vi "Bundle control and indicator references.vi"(8 "error in":errorcluster, 11 "UI elements cluster":T1) -> (0 "error out":errorcluster, 3 "UI elements cluster":T1)   [LabVIEW 2013]
uses:
  Typedefs/UI ctrl refs cluster.ctl
  Typedefs/Laser control knob.ctl
  Typedefs/Frame Size.ctl
  Typedefs/Plane Mode.ctl
  Typedefs/PMT control knob.ctl
  Global Variables/gl_UI Ctrl Refs.vi
panel:
  out "Ctrl ref names in typedef cluster":string[](array[string])
  out "Dynamically acquired UI element names":string[](array[string])
  out "IP same as OP?":T2
  out "Errors":errorcluster[](array[cluster])
  out "UI element names and status":cluster{"Label.Text":string, "Found":bool}[](array[cluster])
  # "<----- If the LED is off for a UI element it means that that this VI fails to acquire its reference correctly. In that case upgrade this VI to handle that element."
  # "The top 5 should be the same.\nThe rest should be updated so not the same."
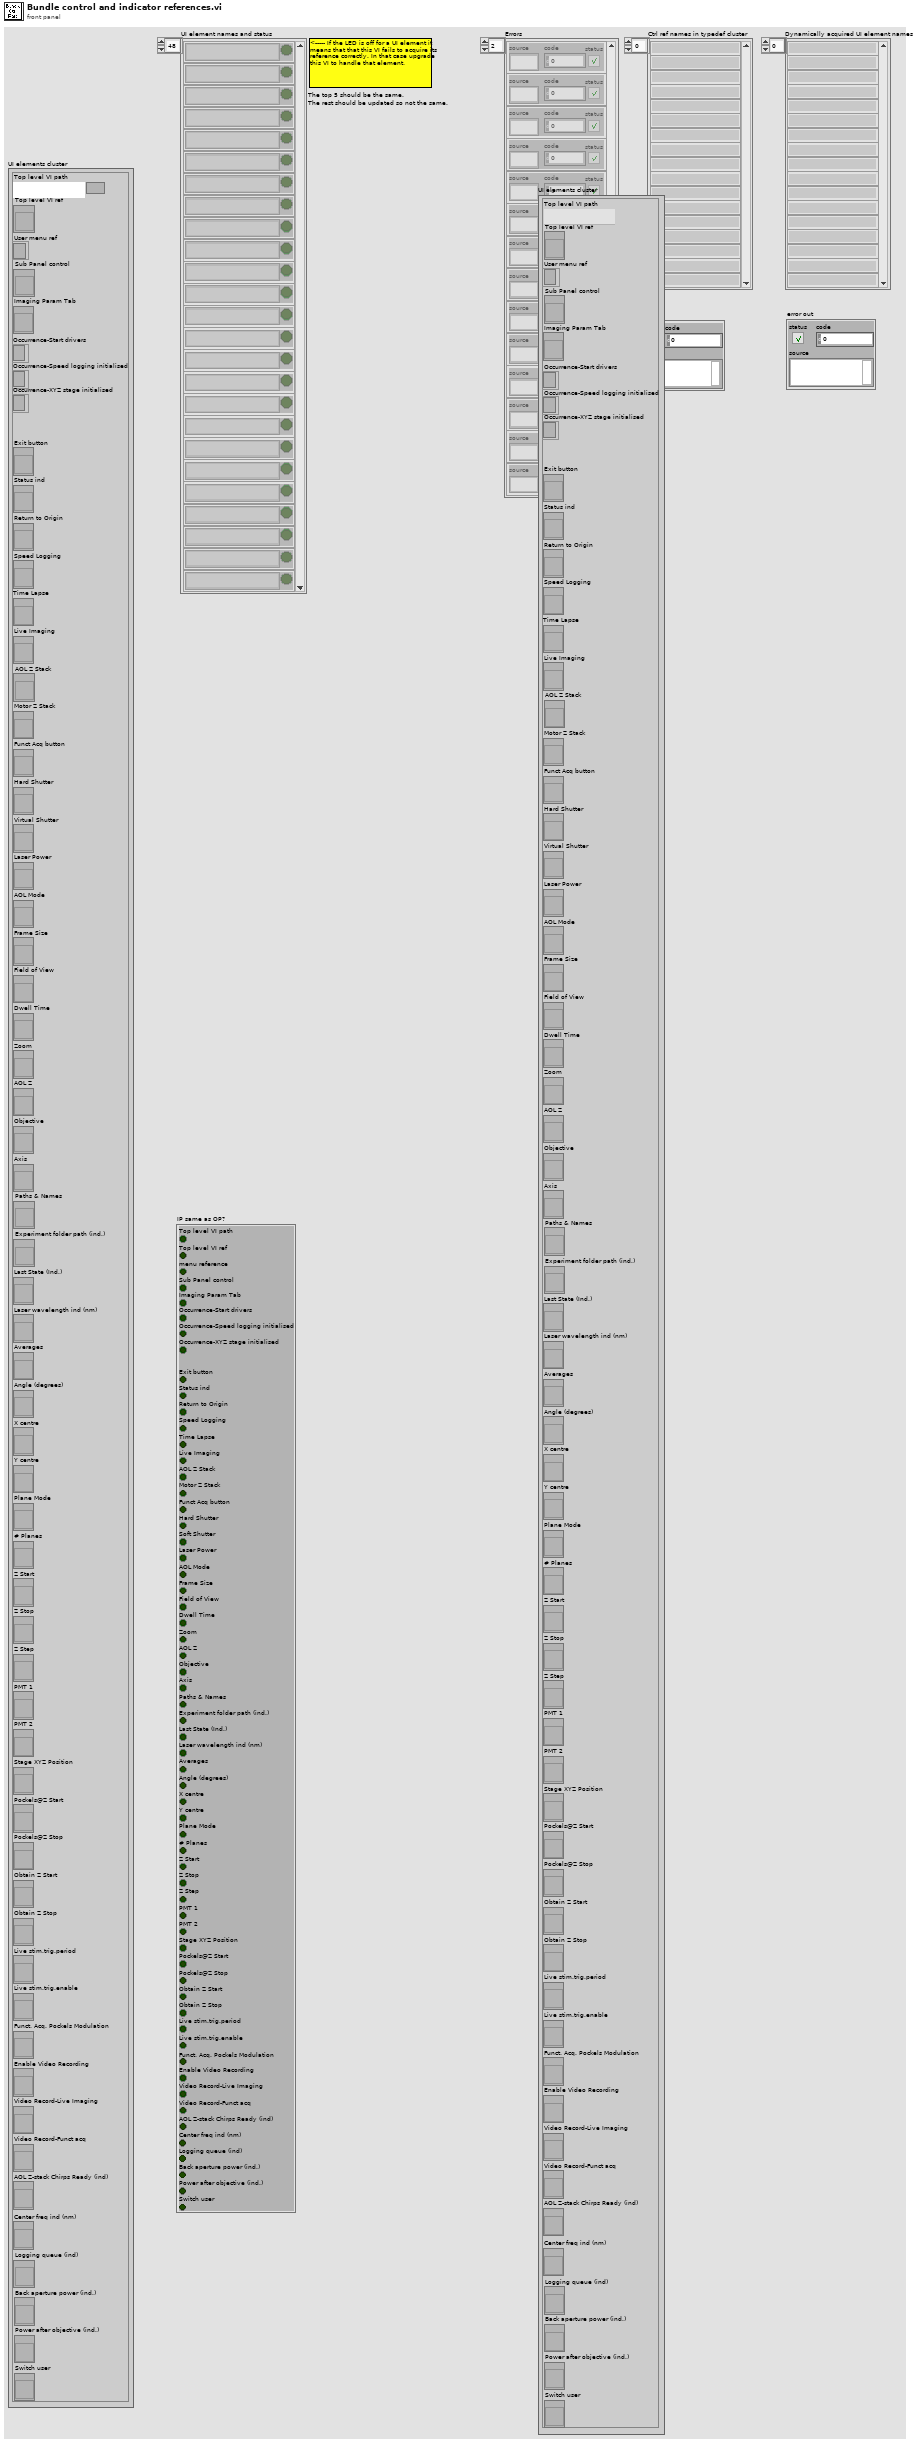
[diagram p1: front panel]
types:
  T1 = typedef "UI ctrl refs cluster.ctl" = cluster{"Top level VI path":path, "Top level VI ref":refnum<vi>, "User menu ref":refnum<k9>, "Sub Panel control":refnum<vi>, "Imaging Param Tab":refnum<vi>, "Occurrence-Start drivers":refnum<k4>, "Occurrence-Speed logging initialised":refnum<k4>, "Occurrence-XYZ stage initialised":refnum<k4>, "Exit button":refnum<vi>, "Status ind":refnum<vi>, "Return to Origin":refnum<vi>, "Speed Logging":refnum<vi>, "Time Lapse":refnum<vi>, "Live Imaging":refnum<vi>, "AOL Z Stack":refnum<vi>, "Motor Z Stack":refnum<vi>, "Funct Acq button":refnum<vi>, "Hard Shutter":refnum<vi>, "Virtual Shutter":refnum<vi>, "Laser Power":refnum<vi>, "AOL Mode":refnum<vi>, "Frame Size":refnum<vi>, "Field of View":refnum<vi>, "Dwell Time":refnum<vi>, "Zoom":refnum<vi>, "AOL Z":refnum<vi>, "Objective":refnum<vi>, "Axis":refnum<vi>, "Paths & Names":refnum<vi>, "Experiment folder path (ind.)":refnum<vi>, "Last State (Ind.)":refnum<vi>, "Laser wavelength ind (nm)":refnum<vi>, "Averages":refnum<vi>, "Angle (degrees)":refnum<vi>, "X centre":refnum<vi>, "Y centre":refnum<vi>, "Plane Mode":refnum<vi>, "# Planes":refnum<vi>, "Z Start":refnum<vi>, "Z Stop":refnum<vi>, "Z Step":refnum<vi>, "PMT 1":refnum<vi>, "PMT 2":refnum<vi>, "Stage XYZ Position":refnum<vi>, "Pockels@Z Start":refnum<vi>, "Pockels@Z Stop":refnum<vi>, "Obtain Z Start":refnum<vi>, "Obtain Z Stop":refnum<vi>, "Live stim.trig.period":refnum<vi>, "Live stim.trig.enable":refnum<vi>, "Funct. Acq. Pockels Modulation":refnum<vi>, "Enable Video Recording":refnum<vi>, "Video Record-Live Imaging":refnum<vi>, "Video Record-Funct acq":refnum<vi>, "AOL Z-stack Chirps Ready (ind)":refnum<vi>, "Center freq ind (nm)":refnum<vi>, "Logging queue (ind)":refnum<vi>, "Back aperture power (ind.)":refnum<vi>, "Power after objective (ind.)":refnum<vi>, "Switch user":refnum<vi>}
  T2 = cluster{"Top level VI path":bool, "Top level VI ref":bool, "menu reference":bool, "Sub Panel control":bool, "Imaging Param Tab":bool, "Occurrence-Start drivers":bool, "Occurrence-Speed logging initialised":bool, "Occurrence-XYZ stage initialised":bool, "Exit button":bool, "Status ind":bool, "Return to Origin":bool, "Speed Logging":bool, "Time Lapse":bool, "Live Imaging":bool, "AOL Z Stack":bool, "Motor Z Stack":bool, "Funct Acq button":bool, "Hard Shutter":bool, "Soft Shutter":bool, "Laser Power":bool, "AOL Mode":bool, "Frame Size":bool, "Field of View":bool, "Dwell Time":bool, "Zoom":bool, "AOL Z":bool, "Objective":bool, "Axis":bool, "Paths & Names":bool, "Experiment folder path (ind.)":bool, "Last State (Ind.)":bool, "Laser wavelength ind (nm)":bool, "Averages":bool, "Angle (degrees)":bool, "X centre":bool, "Y centre":bool, "Plane Mode":bool, "# Planes":bool, "Z Start":bool, "Z Stop":bool, "Z Step":bool, "PMT 1":bool, "PMT 2":bool, "Stage XYZ Position":bool, "Pockels@Z Start":bool, "Pockels@Z Stop":bool, "Obtain Z Stop":bool, "Obtain Z Start":bool, "Live stim.trig.period":bool, "Live stim.trig.enable":bool, "Funct. Acq. Pockels Modulation":bool, "Enable Video Recording":bool, "Video Record-Live Imaging":bool, "Video Record-Funct acq":bool, "AOL Z-stack Chirps Ready (ind)":bool, "Center freq ind (nm)":bool, "Logging queue (ind)":bool, "Back aperture power (ind.)":bool, "Power after objective (ind.)":bool, "Switch user":bool}
  T3 = cluster{"Top level VI path":bool, "Top level VI ref":bool, "User menu ref":bool, "Sub Panel control":bool, "Imaging Param Tab":bool, "Occurrence-Start drivers":bool, "Occurrence-Speed logging initialised":bool, "Occurrence-XYZ stage initialised":bool, "Exit button":bool, "Status ind":bool, "Return to Origin":bool, "Speed Logging":bool, "Time Lapse":bool, "Live Imaging":bool, "AOL Z Stack":bool, "Motor Z Stack":bool, "Funct Acq button":bool, "Hard Shutter":bool, "Virtual Shutter":bool, "Laser Power":bool, "AOL Mode":bool, "Frame Size":bool, "Field of View":bool, "Dwell Time":bool, "Zoom":bool, "AOL Z":bool, "Objective":bool, "Axis":bool, "Paths & Names":bool, "Experiment folder path (ind.)":bool, "Last State (Ind.)":bool, "Laser wavelength ind (nm)":bool, "Averages":bool, "Angle (degrees)":bool, "X centre":bool, "Y centre":bool, "Plane Mode":bool, "# Planes":bool, "Z Start":bool, "Z Stop":bool, "Z Step":bool, "PMT 1":bool, "PMT 2":bool, "Stage XYZ Position":bool, "Pockels@Z Start":bool, "Pockels@Z Stop":bool, "Obtain Z Start":bool, "Obtain Z Stop":bool, "Live stim.trig.period":bool, "Live stim.trig.enable":bool, "Funct. Acq. Pockels Modulation":bool, "Enable Video Recording":bool, "Video Record-Live Imaging":bool, "Video Record-Funct acq":bool, "AOL Z-stack Chirps Ready (ind)":bool, "Center freq ind (nm)":bool, "Logging queue (ind)":bool, "Back aperture power (ind.)":bool, "Power after objective (ind.)":bool, "Switch user":bool}
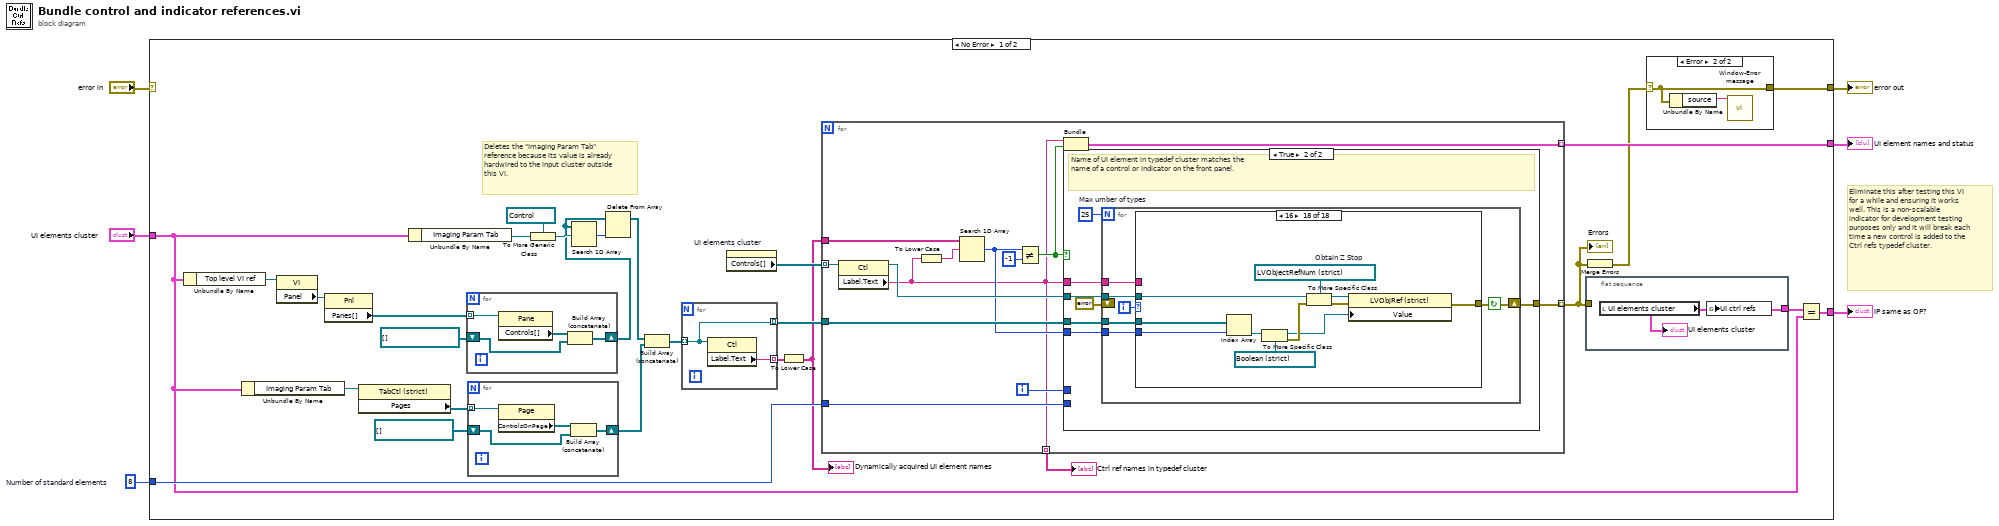
[diagram p0: block diagram]
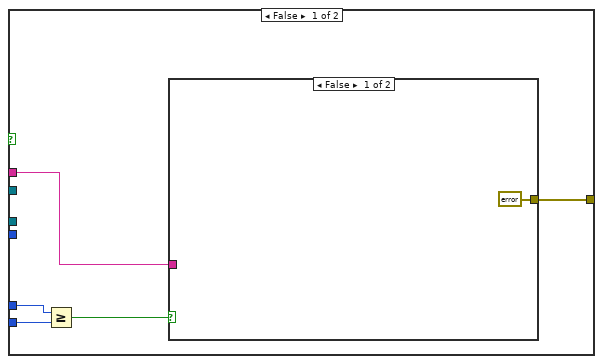
[diagram p3: hidden frame]
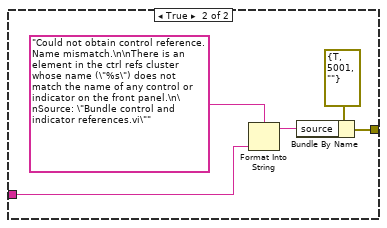
[diagram p4: hidden frame]
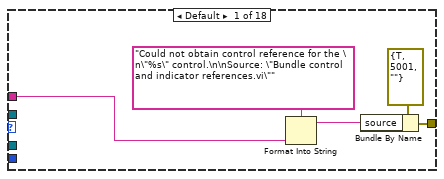
[diagram p5: hidden frame]
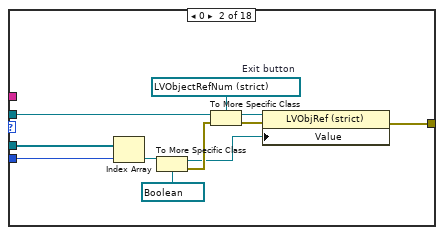
[diagram p6: hidden frame]
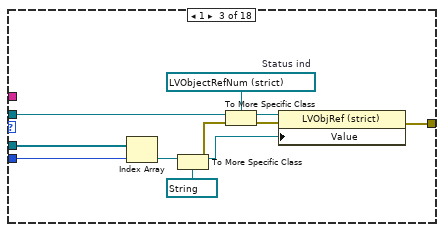
[diagram p7: hidden frame]
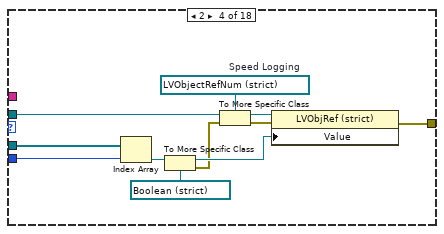
[diagram p8: hidden frame]
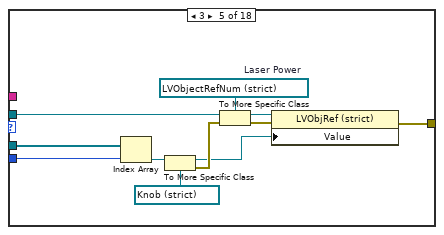
[diagram p9: hidden frame]
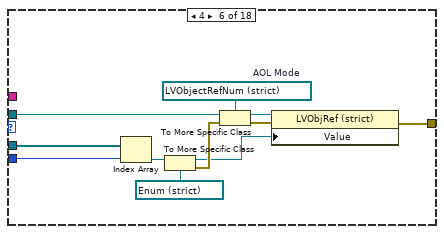
[diagram p10: hidden frame]
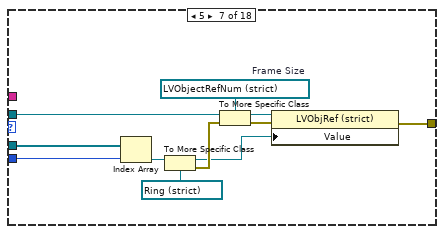
[diagram p11: hidden frame]
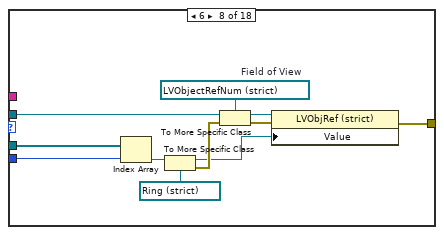
[diagram p12: hidden frame]
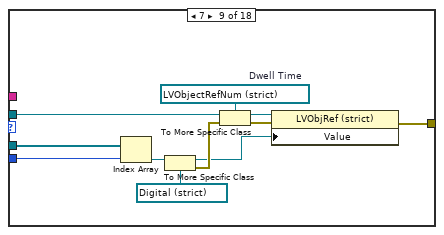
[diagram p13: hidden frame]
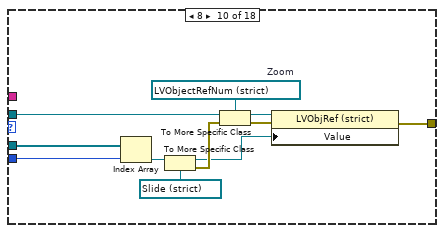
[diagram p14: hidden frame]
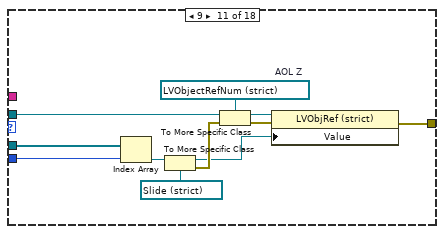
[diagram p15: hidden frame]
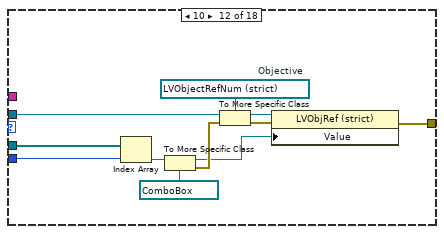
[diagram p16: hidden frame]
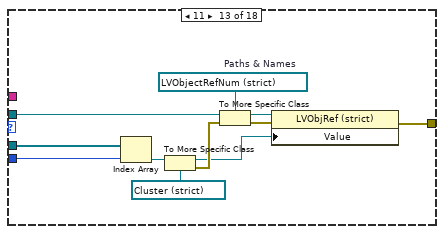
[diagram p17: hidden frame]
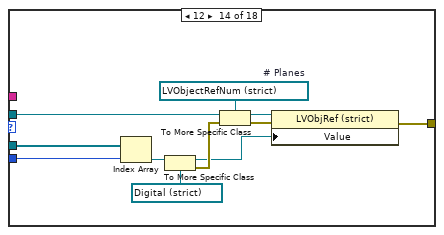
[diagram p18: hidden frame]
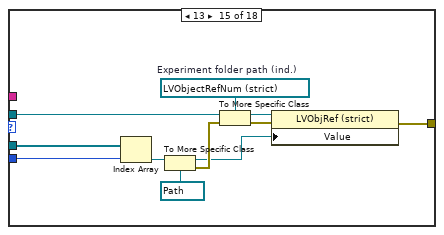
[diagram p19: hidden frame]
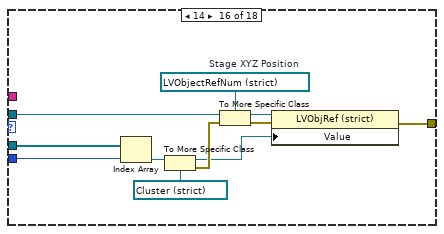
[diagram p20: hidden frame]
diagram:
  w2 = 8  # Number of standard elements
  # "Eliminate this after testing this VI for a while and ensuring it works well. This is a non-scalable indicator for development testing purposes only and it will break each time a new control is added to the Ctrl refs typedef cluster."
  n1 = case shown="No Error" "error in" {
    selector: "error in" -> [_ w277]
    tunnel: [w24 _] -> w6
    tunnel: "UI elements cluster" -> [w10 _]
    tunnel: [w22 _] -> w1
    tunnel: [w13 w277] -> w3
    tunnel: w2 -> [w12 _]
    frame No Error {
      # "Deletes the \"Imaging Param Tab\" reference because its value is already hardwired to the input cluster outside this VI."
      n2 = Unbundle By Name(w10) -> ("Top level VI ref"=w33:refnum<vi>)
      n3 = Unbundle By Name(w10) -> ("Imaging Param Tab"=w19:refnum<vi>)
      n4 = property on="Property Node" class="VI"(reference=w33) -> ("Panel"=w34:refnum<vi>)  [unwired: 1 in, 2 out]
      n5 = property on="Property Node" class="Pnl"(reference=w34) -> ("Panes[]"=w31:refnum<vi>[])  [unwired: 1 in, 2 out]
      n6 = property on="Property Node" class="TabCtl (strict)"(reference=w19) -> ("Pages"=w30:refnum<vi>[])  [unwired: 1 in, 2 out]
      n7 = Unbundle By Name(w10) -> ("Imaging Param Tab"=w11:refnum<vi>)
      n8 = for {
        shift-right: [w275] -> w9
        shift-left: refnum<vi>[] [] -> [w274]
        tunnel: w31 -> [w273] mode=indexing
        n9 = property class="Pane"(reference=w273) -> ("Controls[]"=w276:refnum<vi>[])  [unwired: 1 in, 2 out]
        n10 = Build Array (concatenate)(w276, w274) -> (w275:refnum<vi>[])
      }
      n11 = for {
        shift-right: [w269] -> w28
        shift-left: refnum<vi>[] [] -> [w268]
        tunnel: w30 -> [w267] mode=indexing
        n12 = property class="Page"(reference=w267) -> ("ControlsOnPage"=w270:refnum<vi>[])  [unwired: 1 in, 2 out]
        n13 = Build Array (concatenate)(w270, w268) -> (w269:refnum<vi>[])
      }
      n14 = To More Generic Class(target class=refnum<vi> refnum ("element"), reference=w11) -> (generic class reference=w18:refnum<vi>)
      n15 = Search 1D Array(1D array=w9, element=w18) -> (index of element=w16:i32)  [unwired: 1 in]
      n16 = Delete From Array(array=w9, index=w16) -> (array with subset deleted=w15:refnum<vi>[])  [unwired: 1 in, 1 out]
      n17 = Build Array (concatenate)(w15, w28) -> (w27:refnum<vi>[])
      n18 = for {
        tunnel: w27 -> [w271] mode=indexing
        tunnel: [w272] -> w25 mode=indexing
        tunnel: [w271] -> w23 mode=indexing
        n19 = property on="Property Node" class="Ctl"(reference=w271) -> ("Label.Text"=w272:string)  [unwired: 1 in, 2 out]
      }
      n20 = property on="UI elements cluster" class="Clust (strict)"() -> ("Controls[]"=w26:refnum<vi>[])  [unwired: 2 in, 2 out]
      n21 = To Lower Case(string=w25) -> (all lower case string=w8:string[])
      "Dynamically acquired UI element names" <- w8
      n22 = for {
        tunnel: w26 -> [w50] mode=indexing
        tunnel: w8 -> [w49]
        tunnel: [w47] -> w24 mode=indexing
        tunnel: [w45] -> w21 mode=indexing
        tunnel: w23 -> [w43]
        tunnel: w12 -> [w40]
        tunnel: [w38] -> w7 mode=indexing
        i -> [w41]
        n23 = property on="Property Node" class="Ctl"(reference=w50) -> (reference out=w46:refnum<vi>, "Label.Text"=w38:string)  [unwired: 1 in, 1 out]
        n24 = To Lower Case(string=w38) -> (all lower case string=w42:string)
        n25 = Search 1D Array(1D array=w49, element=w42) -> (index of element=w39:i32)  [unwired: 1 in]
        n26 = Not Equal?(x=w39, y=-1) -> (x != y?=w44:bool)
        n27 = Bundle("Label.Text"=w38, w44) -> (w47:cluster{"Label.Text":string, bool})  [unwired: 1 in]
        n28 = case shown="True" w44 {
          tunnel: w46 -> [_ w68]
          tunnel: [w53 w67] -> w45
          tunnel: w43 -> [_ w66]
          tunnel: w39 -> [_ w65]
          tunnel: w38 -> [w51 w62]
          tunnel: w41 -> [w55 _]
          tunnel: w40 -> [w52 _]
          frame False {
            n29 = Greater Or Equal?(x=w55, y=w52) -> (x >= y?=w54:bool)
            n30 = case shown="False" w54 {
              tunnel: [errorcluster {"status"=FALSE, "code"=0, "source"=""} ("error out") w60] -> w53
              tunnel: w51 -> [_ w57]
              frame False {
              }
              frame True {
                n31 = Format Into String(format string="Could not obtain control reference. Name mismatch.\n\nThere is an element in the ctrl refs cluster whose name (\"%s\") does not match the name of any control or indicator on the front panel.\n\nSource: \"Bundle control and indicator references.vi\"" ("source"), w57) -> (resulting string=w59:string)  [unwired: 2 in, 1 out]
                n32 = Bundle By Name(cluster=errorcluster {"status"=TRUE, "code"=5001, "source"=""} ("error out"), "source"=w59) -> (w60:errorcluster)
              }
            }
          }
          frame True {
            w64 = 25  # Max umber of types
            # "Name of UI element in typedef cluster matches the\nname of a control or indicator on the front panel."
            n33 = for {
              N: w64 -> [_]
              tunnel: w68 -> [w74]
              tunnel: w66 -> [w73]
              tunnel: w65 -> [w72]
              shift-right: [w70] -> w67
              shift-left: errorcluster {"status"=FALSE, "code"=0, "source"=""} ("error out") -> [_]
              tunnel: w62 -> [w69]
              i -> [w71]
              stop <- w70 continue-if-true
              n34 = case shown="16" w71 {
                tunnel: w74 -> [_ w86 w101 w112 w123 w134 w145 w156 w167 w178 w189 w200 w211 w222 w233 w244 w255 w266]
                tunnel: [w78 w83 w100 w109 w119 w130 w141 w152 w163 w174 w185 w196 w207 w218 w229 w240 w251 w262] -> w70
                tunnel: w73 -> [_ w84 w99 w111 w122 w133 w144 w155 w166 w177 w188 w199 w210 w221 w232 w243 w254 w265]
                tunnel: w72 -> [_ w85 w98 w110 w121 w132 w143 w154 w165 w176 w187 w198 w209 w220 w231 w242 w253 w264]
                tunnel: w69 -> [w76 _ _ _ _ _ _ _ _ _ _ _ _ _ _ _ _ _]
                frame Default {
                  n35 = Format Into String(format string="Could not obtain control reference for the \n\"%s\" control.\n\nSource: \"Bundle control and indicator references.vi\"" ("source"), w76) -> (resulting string=w75:string)  [unwired: 2 in, 1 out]
                  n36 = Bundle By Name(cluster=errorcluster {"status"=TRUE, "code"=5001, "source"=""} ("error out"), "source"=w75) -> (w78:errorcluster)
                }
                frame 0 {
                  w80 = refnum<vi> refnum  # Exit button
                  n37 = Index Array(array=w84, index=w85) -> (element=w89:refnum<vi>)
                  n38 = To More Specific Class(target class=refnum<vi> refnum ("Value"), reference=w89) -> (specific class reference=w81:refnum<vi>, error out=w88:errorcluster)  [unwired: 1 in]
                  n39 = To More Specific Class(target class=w80, reference=w86, error in=w88) -> (specific class reference=w90:refnum<vi>, error out=w87:errorcluster)
                  n40 = property on="Property Node" class="LVObjRef (strict)"(reference=w90, error in=w87, "Value"=w81) -> (error out=w83:errorcluster)  [unwired: 1 out]
                }
                frame 1 {
                  w91 = refnum<vi> refnum  # Status ind
                  n41 = Index Array(array=w99, index=w98) -> (element=w96:refnum<vi>)
                  n42 = To More Specific Class(target class=refnum<vi> refnum ("Status ind"), reference=w96) -> (specific class reference=w95:refnum<vi>, error out=w94:errorcluster)  [unwired: 1 in]
                  n43 = To More Specific Class(target class=w91, reference=w101, error in=w94) -> (specific class reference=w97:refnum<vi>, error out=w93:errorcluster)
                  n44 = property on="Property Node" class="LVObjRef (strict)"(reference=w97, error in=w93, "Value"=w95) -> (error out=w100:errorcluster)  [unwired: 1 out]
                }
                frame 2 {
                  w102 = refnum<vi> refnum  # Speed Logging
                  n45 = Index Array(array=w111, index=w110) -> (element=w108:refnum<vi>)
                  n46 = To More Specific Class(target class=refnum<vi> refnum ("Value"), reference=w108) -> (specific class reference=w107:refnum<vi>, error out=w104:errorcluster)  [unwired: 1 in]
                  n47 = To More Specific Class(target class=w102, reference=w112, error in=w104) -> (specific class reference=w106:refnum<vi>, error out=w105:errorcluster)
                  n48 = property on="Property Node" class="LVObjRef (strict)"(reference=w106, error in=w105, "Value"=w107) -> (error out=w109:errorcluster)  [unwired: 1 out]
                }
                frame 3 {
                  w113 = refnum<vi> refnum  # Laser Power
                  n49 = Index Array(array=w122, index=w121) -> (element=w120:refnum<vi>)
                  n50 = To More Specific Class(target class=refnum<vi> refnum ("Value"), reference=w120) -> (specific class reference=w114:refnum<vi>, error out=w116:errorcluster)  [unwired: 1 in]
                  n51 = To More Specific Class(target class=w113, reference=w123, error in=w116) -> (specific class reference=w118:refnum<vi>, error out=w117:errorcluster)
                  n52 = property on="Property Node" class="LVObjRef (strict)"(reference=w118, error in=w117, "Value"=w114) -> (error out=w119:errorcluster)  [unwired: 1 out]
                }
                frame 4 {
                  w124 = refnum<vi> refnum  # AOL Mode
                  n53 = Index Array(array=w133, index=w132) -> (element=w131:refnum<vi>)
                  n54 = To More Specific Class(target class=refnum<vi> refnum ("Value"), reference=w131) -> (specific class reference=w126:refnum<vi>, error out=w127:errorcluster)  [unwired: 1 in]
                  n55 = To More Specific Class(target class=w124, reference=w134, error in=w127) -> (specific class reference=w129:refnum<vi>, error out=w128:errorcluster)
                  n56 = property on="Property Node" class="LVObjRef (strict)"(reference=w129, error in=w128, "Value"=w126) -> (error out=w130:errorcluster)  [unwired: 1 out]
                }
                frame 5 {
                  w135 = refnum<vi> refnum  # Frame Size
                  n57 = Index Array(array=w144, index=w143) -> (element=w142:refnum<vi>)
                  n58 = To More Specific Class(target class=refnum<vi> refnum ("Value"), reference=w142) -> (specific class reference=w136:refnum<vi>, error out=w138:errorcluster)  [unwired: 1 in]
                  n59 = To More Specific Class(target class=w135, reference=w145, error in=w138) -> (specific class reference=w140:refnum<vi>, error out=w139:errorcluster)
                  n60 = property on="Property Node" class="LVObjRef (strict)"(reference=w140, error in=w139, "Value"=w136) -> (error out=w141:errorcluster)  [unwired: 1 out]
                }
                frame 6 {
                  w146 = refnum<vi> refnum  # Field of View
                  n61 = Index Array(array=w155, index=w154) -> (element=w153:refnum<vi>)
                  n62 = To More Specific Class(target class=refnum<vi> refnum ("Value"), reference=w153) -> (specific class reference=w148:refnum<vi>, error out=w149:errorcluster)  [unwired: 1 in]
                  n63 = To More Specific Class(target class=w146, reference=w156, error in=w149) -> (specific class reference=w151:refnum<vi>, error out=w150:errorcluster)
                  n64 = property on="Property Node" class="LVObjRef (strict)"(reference=w151, error in=w150, "Value"=w148) -> (error out=w152:errorcluster)  [unwired: 1 out]
                }
                frame 7 {
                  w157 = refnum<vi> refnum  # Dwell Time
                  n65 = Index Array(array=w166, index=w165) -> (element=w164:refnum<vi>)
                  n66 = To More Specific Class(target class=refnum<vi> refnum ("Value"), reference=w164) -> (specific class reference=w159:refnum<vi>, error out=w160:errorcluster)  [unwired: 1 in]
                  n67 = To More Specific Class(target class=w157, reference=w167, error in=w160) -> (specific class reference=w162:refnum<vi>, error out=w161:errorcluster)
                  n68 = property on="Property Node" class="LVObjRef (strict)"(reference=w162, error in=w161, "Value"=w159) -> (error out=w163:errorcluster)  [unwired: 1 out]
                }
                frame 8 {
                  w168 = refnum<vi> refnum  # Zoom
                  n69 = Index Array(array=w177, index=w176) -> (element=w175:refnum<vi>)
                  n70 = To More Specific Class(target class=refnum<vi> refnum ("Value"), reference=w175) -> (specific class reference=w170:refnum<vi>, error out=w171:errorcluster)  [unwired: 1 in]
                  n71 = To More Specific Class(target class=w168, reference=w178, error in=w171) -> (specific class reference=w173:refnum<vi>, error out=w172:errorcluster)
                  n72 = property on="Property Node" class="LVObjRef (strict)"(reference=w173, error in=w172, "Value"=w170) -> (error out=w174:errorcluster)  [unwired: 1 out]
                }
                frame 9 {
                  w179 = refnum<vi> refnum  # AOL Z
                  n73 = Index Array(array=w188, index=w187) -> (element=w186:refnum<vi>)
                  n74 = To More Specific Class(target class=refnum<vi> refnum ("Value"), reference=w186) -> (specific class reference=w181:refnum<vi>, error out=w182:errorcluster)  [unwired: 1 in]
                  n75 = To More Specific Class(target class=w179, reference=w189, error in=w182) -> (specific class reference=w184:refnum<vi>, error out=w183:errorcluster)
                  n76 = property on="Property Node" class="LVObjRef (strict)"(reference=w184, error in=w183, "Value"=w181) -> (error out=w185:errorcluster)  [unwired: 1 out]
                }
                frame 10 {
                  w190 = refnum<vi> refnum  # Objective
                  n77 = Index Array(array=w199, index=w198) -> (element=w197:refnum<vi>)
                  n78 = To More Specific Class(target class=refnum<vi> refnum ("Value"), reference=w197) -> (specific class reference=w192:refnum<vi>, error out=w193:errorcluster)  [unwired: 1 in]
                  n79 = To More Specific Class(target class=w190, reference=w200, error in=w193) -> (specific class reference=w195:refnum<vi>, error out=w194:errorcluster)
                  n80 = property on="Property Node" class="LVObjRef (strict)"(reference=w195, error in=w194, "Value"=w192) -> (error out=w196:errorcluster)  [unwired: 1 out]
                }
                frame 11 {
                  w202 = refnum<vi> refnum  # Paths & Names
                  n81 = Index Array(array=w210, index=w209) -> (element=w208:refnum<vi>)
                  n82 = To More Specific Class(target class=refnum<vi> refnum ("Paths & Names"), reference=w208) -> (specific class reference=w203:refnum<vi>, error out=w204:errorcluster)  [unwired: 1 in]
                  n83 = To More Specific Class(target class=w202, reference=w211, error in=w204) -> (specific class reference=w206:refnum<vi>, error out=w205:errorcluster)
                  n84 = property on="Property Node" class="LVObjRef (strict)"(reference=w206, error in=w205, "Value"=w203) -> (error out=w207:errorcluster)  [unwired: 1 out]
                }
                frame 12 {
                  w212 = refnum<vi> refnum  # # Planes
                  n85 = Index Array(array=w221, index=w220) -> (element=w219:refnum<vi>)
                  n86 = To More Specific Class(target class=refnum<vi> refnum ("Value"), reference=w219) -> (specific class reference=w214:refnum<vi>, error out=w215:errorcluster)  [unwired: 1 in]
                  n87 = To More Specific Class(target class=w212, reference=w222, error in=w215) -> (specific class reference=w217:refnum<vi>, error out=w216:errorcluster)
                  n88 = property on="Property Node" class="LVObjRef (strict)"(reference=w217, error in=w216, "Value"=w214) -> (error out=w218:errorcluster)  [unwired: 1 out]
                }
                frame 13 {
                  w224 = refnum<vi> refnum  # Experiment folder path (ind.)
                  n89 = Index Array(array=w232, index=w231) -> (element=w230:refnum<vi>)
                  n90 = To More Specific Class(target class=refnum<vi> refnum ("Experiment folder path (ind.)"), reference=w230) -> (specific class reference=w225:refnum<vi>, error out=w226:errorcluster)  [unwired: 1 in]
                  n91 = To More Specific Class(target class=w224, reference=w233, error in=w226) -> (specific class reference=w228:refnum<vi>, error out=w227:errorcluster)
                  n92 = property on="Property Node" class="LVObjRef (strict)"(reference=w228, error in=w227, "Value"=w225) -> (error out=w229:errorcluster)  [unwired: 1 out]
                }
                frame 14 {
                  w234 = refnum<vi> refnum  # Stage XYZ Position
                  n93 = Index Array(array=w243, index=w242) -> (element=w241:refnum<vi>)
                  n94 = To More Specific Class(target class=refnum<vi> refnum ("Value"), reference=w241) -> (specific class reference=w236:refnum<vi>, error out=w237:errorcluster)  [unwired: 1 in]
                  n95 = To More Specific Class(target class=w234, reference=w244, error in=w237) -> (specific class reference=w239:refnum<vi>, error out=w238:errorcluster)
                  n96 = property on="Property Node" class="LVObjRef (strict)"(reference=w239, error in=w238, "Value"=w236) -> (error out=w240:errorcluster)  [unwired: 1 out]
                }
                frame 15 {
                  w245 = refnum<vi> refnum  # Pockels@Z Stop
                  n97 = Index Array(array=w254, index=w253) -> (element=w252:refnum<vi>)
                  n98 = To More Specific Class(target class=refnum<vi> refnum ("Value"), reference=w252) -> (specific class reference=w247:refnum<vi>, error out=w248:errorcluster)  [unwired: 1 in]
                  n99 = To More Specific Class(target class=w245, reference=w255, error in=w248) -> (specific class reference=w250:refnum<vi>, error out=w249:errorcluster)
                  n100 = property on="Property Node" class="LVObjRef (strict)"(reference=w250, error in=w249, "Value"=w247) -> (error out=w251:errorcluster)  [unwired: 1 out]
                }
                frame 16 {
                  w256 = refnum<vi> refnum  # Obtain Z Stop
                  n101 = Index Array(array=w265, index=w264) -> (element=w263:refnum<vi>)
                  n102 = To More Specific Class(target class=refnum<vi> refnum ("Value"), reference=w263) -> (specific class reference=w257:refnum<vi>, error out=w259:errorcluster)  [unwired: 1 in]
                  n103 = To More Specific Class(target class=w256, reference=w266, error in=w259) -> (specific class reference=w261:refnum<vi>, error out=w260:errorcluster)
                  n104 = property on="Property Node" class="LVObjRef (strict)"(reference=w261, error in=w260, "Value"=w257) -> (error out=w262:errorcluster)  [unwired: 1 out]
                }
              }
            }
          }
        }
      }
      "Errors" <- w21
      "Ctrl ref names in typedef cluster" <- w7
      n105 = flat-sequence {
        tunnel: w21 -> [_]
        tunnel: [w37] -> w20
        frame #0 {
          n106 = local read "UI elements cluster"() -> (w37:T1)
          "UI elements cluster" <- w37
          n107 = global write "gl_UI Ctrl Refs.vi" "UI ctrl refs"(w37) -> ()
        }
      }
      n108 = Merge Errors(w21) -> (w14:errorcluster)
      n109 = case shown="Error" w14 {
        selector: w14 -> [_ w36]
        tunnel: [_ w36] -> w13
        frame No Error {
        }
        frame Error {
          n110 = Unbundle By Name(w36) -> ("source"=w35:string)
          n111 = call "Window-Error message.vi"("Message"=w35) -> ()  [unwired: 10 in, 1 out]
        }
      }
      n112 = Equal?(x=w20, y=w10) -> (x = y?=w22:T3)
    }
    frame Error {
    }
  }
  "error out" <- w3
  "UI element names and status" <- w6
  "IP same as OP?" <- w1
